vi "cumsum_dQ.vi"(1 "index start cumsum\n(zeros before)":i32, 2 "Enc. res. [CAD/sample]":dbl=0.1 format="%#_13g", 3 "dQ":dbl[](array[numeric])) -> (0 "Qcum":dbl[](array[numeric]))   [LabVIEW 2020]
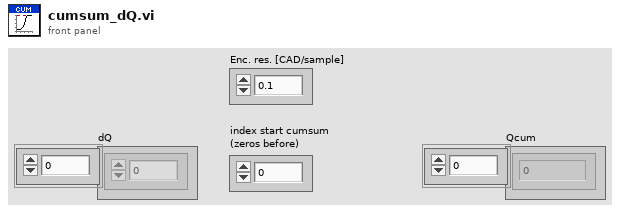
[diagram p1: front panel]
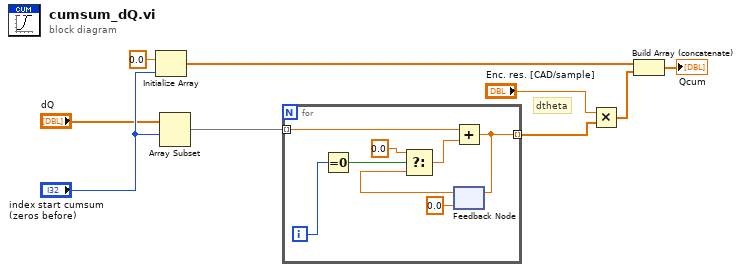
[diagram p0: block diagram]
diagram:
  # "dtheta"
  n1 = Initialize Array(0.0 ("element"), "index start cumsum\n(zeros before)") -> (w6:dbl[])
  n2 = Array Subset(array="dQ", index="index start cumsum\n(zeros before)") -> (w8:dbl[])  [unwired: 1 in]
  n3 = for {
    tunnel: w8 -> [w17] mode=indexing
    tunnel: [w15] -> w7 mode=indexing
    i -> [w12]
    n4 = Equal To 0?(x=w12) -> (x = 0?=w13:bool)
    n5 = feedback #1(0.0) -> (w11:dbl)
    n6 = Select(t=0.0, s=w13, f=w11) -> (s? t:f=w14:dbl)
    n7 = Add(x=w17, y=w14) -> (x+y=w15:dbl)
    n8 = feedback-in #1(w15) -> ()
  }
  n9 = Multiply(x="Enc. res. [CAD/sample]", y=w7) -> (x*y=w5:dbl[])
  n10 = Build Array (concatenate)(w6, w5) -> (→"Qcum":dbl[])
